vi "Drive.vi"() -> ()   [LabVIEW 2016]
panel:
  out "Shifter Position":dbl
  out "Right Motor Voltage":dbl
  out "Left Motor Voltage":dbl
  in  "High Gear":bool
  in  "Right Power":dbl
  in  "Left Power":dbl
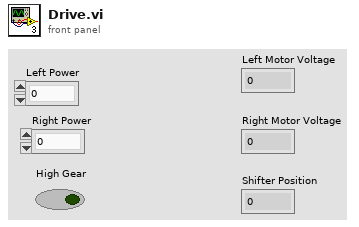
[diagram p1: front panel]
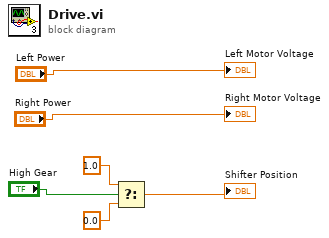
[diagram p0: block diagram]
diagram:
  n1 = Select(t=1.0, s="High Gear", f=0.0) -> (s? t:f=→"Shifter Position":dbl)
  "Left Motor Voltage" <- "Left Power"
  "Right Motor Voltage" <- "Right Power"
